vi "ClusterEscala.vi"() -> ()   [LabVIEW 2020]
panel:
  out "x*y":cluster{dbl, dbl, dbl} {"?" scale=0.0..100.0; "?" scale=0.0..1000.0; "?" scale=0.0..100.0}
  in  "Cluster 2":T1
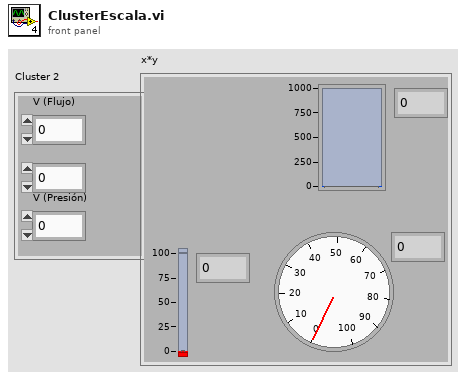
[diagram p1: front panel]
types:
  T1 = cluster{"V (Temperatura)":dbl, "V (Flujo)":dbl, "V (Presión)":dbl}
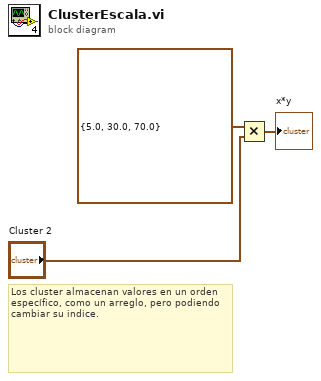
[diagram p0: block diagram]
diagram:
  # "Los cluster almacenan valores en un orden específico, como un arreglo, pero podiendo cambiar su indice."
  n1 = Multiply(x=cluster{dbl, dbl, dbl} {5.0, 30.0, 70.0}, y="Cluster 2") -> (x*y=→"x*y":cluster{dbl, dbl, dbl})
